vi "DSF.Engine.Runtime.Framework.Set Runtime Data.vi"(8 "error in (no error)":errorcluster, 10 "Framework Runtime Data":T1, 11 "Framework Runtime in":refnum<class "DSF.Engine.Runtime.Framework.lvclass">) -> (0 "error out":errorcluster, 3 "Framework Runtime out":refnum<class "DSF.Engine.Runtime.Framework.lvclass">)   [LabVIEW 2016, in "DSF.Engine.lvlib" / "DSF.Engine.Runtime.Framework.lvclass"]
uses:
  DSF.Engine.Runtime.Framework.lvclass
  DSF.Engine.Runtime.Framework.Runtime Data.ctl
  DSF.Engine.Runtime.Framework.lvclass/DSF.Engine.Runtime.Framework.ctl
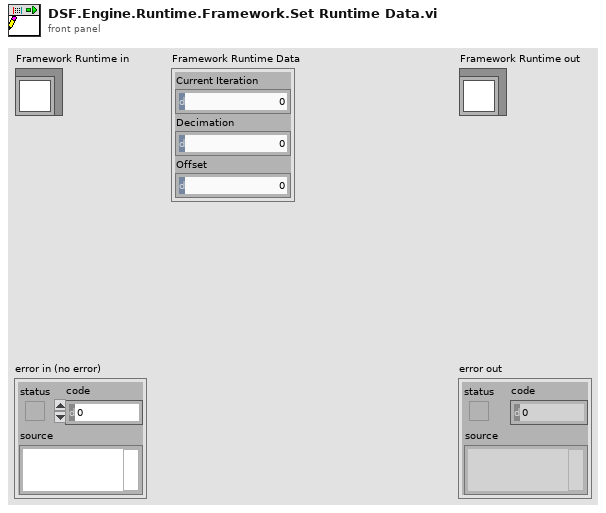
[diagram p1: front panel]
types:
  T1 = typedef "DSF.Engine.lvlib/DSF.Engine.Runtime.Framework.lvclass/DSF.Engine.Runtime.Framework.Runtime Data.ctl" = cluster{"Current Iteration":u64, "Decimation":u64, "Offset":u64}
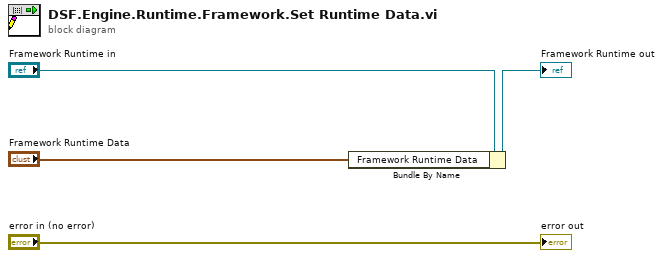
[diagram p0: block diagram]
diagram:
  n1 = Bundle By Name(cluster="Framework Runtime in", "Framework Runtime Data"="Framework Runtime Data") -> (→"Framework Runtime out":refnum<class "DSF.Engine.Runtime.Framework.lvclass">)
  "error out" <- "error in (no error)"
